vi "InitBallHandling.vi"   [LabVIEW 2023]
doc: "This VI initializes miscellaneous devices such as the compressor and any decorations."
uses:
  <vilib>/Rock Robotics/WPI/ThirdParty/Phoenix-LabVIEW/Motor Controller/Controls/CTRE_Phoenix_MotorControl_TalonFXInvertType.ctl
  <vilib>/Rock Robotics/WPI/ThirdParty/Phoenix-LabVIEW/Motor Controller/Controls/CTRE_Phoenix_MotorControl_NeutralMode.ctl
  <vilib>/Rock Robotics/WPI/ThirdParty/Phoenix-LabVIEW/Motor Controller/Controls/CTRE_Phoenix_MotorControl_FeedbackDevice_TalonFX.ctl
  <vilib>/Rock Robotics/WPI/ThirdParty/Phoenix-LabVIEW/Motor Controller/Controls/CTRE_Phoenix_MotorControl_SupplyCurrentLimitConfiguration.ctl
  <vilib>/Rock Robotics/WPI/ThirdParty/Phoenix-LabVIEW/Motor Controller/Controls/CTRE_Phoenix_MotorControl_StatusFrameEnhanced.ctl
  <vilib>/Rock Robotics/WPI/ThirdParty/Phoenix-LabVIEW/Motor Controller/Controls/CTRE_Phoenix_MotorControl_LimitSwitchSource_Local.ctl
  <vilib>/Rock Robotics/WPI/ThirdParty/Phoenix-LabVIEW/Motor Controller/Controls/CTRE_Phoenix_MotorControl_LimitSwitchNormal.ctl
  GlobalBallHandling.vi
types:
  T1 = typedef "CTRE_Phoenix_MotorControl_LimitSwitchNormal.ctl" = enum16{"Normally Open", "Normally Closed", "Disabled"}
  T2 = typedef "CTRE_Phoenix_MotorControl_LimitSwitchSource_Local.ctl" = enum16{"Feedback Connector", "Remote Talon SRX", "Remote CANifier", "Deactivated"}
  T3 = typedef "CTRE_Phoenix_MotorControl_StatusFrameEnhanced.ctl" = u16
  T4 = typedef "CTRE_Phoenix_MotorControl_SupplyCurrentLimitConfiguration.ctl" = cluster{"Enable?":bool, "Current Limit":dbl, "Threshold Current":dbl, "Threshold Time":dbl}
  T5 = typedef "CTRE_Phoenix_MotorControl_FeedbackDevice_TalonFX.ctl" = i8
  T6 = typedef "CTRE_Phoenix_MotorControl_NeutralMode.ctl" = enum8{"EEPROMSetting", "Override to Coast", "Override to Brake"}
  T7 = typedef "CTRE_Phoenix_MotorControl_TalonFXInvertType.ctl" = enum16{"Counter-Clockwise", "Clockwise"}
  T8 = typedef "WPI_MotorControlDeviceRef.ctl" = cluster{"DeviceStatus":errorcluster, "Type":T9, "PWM":cluster{"PWM Channel":T10, "DeadBand":T11}, "CAN":cluster{"Device Number":u8, "SetOutput VI Ref":variant, "GetOutput VI Ref":variant, "Enable VI Ref":variant, "Disable VI Ref":variant, "Data":variant}, "Invert":bool, "DIO PWM":cluster{"PWM \"Enable\" Channel":T10, "DIOChannel":T12, "PWM Rate":dbl}}
  T9 = typedef "WPI_MotorControlType.ctl" = enum16{"PWM", "CAN", "DIO PWM"}
  T10 = typedef "FPGA_DIOPWMChannel.ctl" = enum8{"PWM 0", "PWM 1", "PWM 2", "PWM 3", "PWM 4", "PWM 5", "PWM 6", "PWM 7", "PWM 8", "PWM 9", "PWM MXP 0", "PWM MXP 1", "PWM MXP 2", "PWM MXP 3", "PWM MXP 4", "PWM MXP 5", "PWM MXP 6", "PWM MXP 7", "PWM MXP 8", "PWM MXP 9", "Invalid"}
  T11 = typedef "WPI_PWMDeadband.ctl" = cluster{"Name":string, "maxPositivePwm":i32, "minPositivePwm":i32, "centerPwm":i32, "maxNegativePwm":i32, "minNegativePwm":i32, "angularRange":u16}
  T12 = typedef "FPGA_DIOChannel.ctl" = enum8{"DIO 0", "DIO 1", "DIO 2", "DIO 3", "DIO 4", "DIO 5", "DIO 6", "DIO 7", "DIO 8", "DIO 9", "DIO MXP 0", "DIO MXP 1", "DIO MXP 2", "DIO MXP 3", "DIO MXP 4", "DIO MXP 5", "DIO MXP 6", "DIO MXP 7", "DIO MXP 8", "DIO MXP 9", "DIO MXP 10", "DIO MXP 11", "DIO MXP 12", "DIO MXP 13", "DIO MXP 14", "DIO MXP 15", "SPI Port CS1", "SPI Port CS2", "SPI Port CS3", "SPI Port MISO", "SPI Port MOSI", "Invalid"}
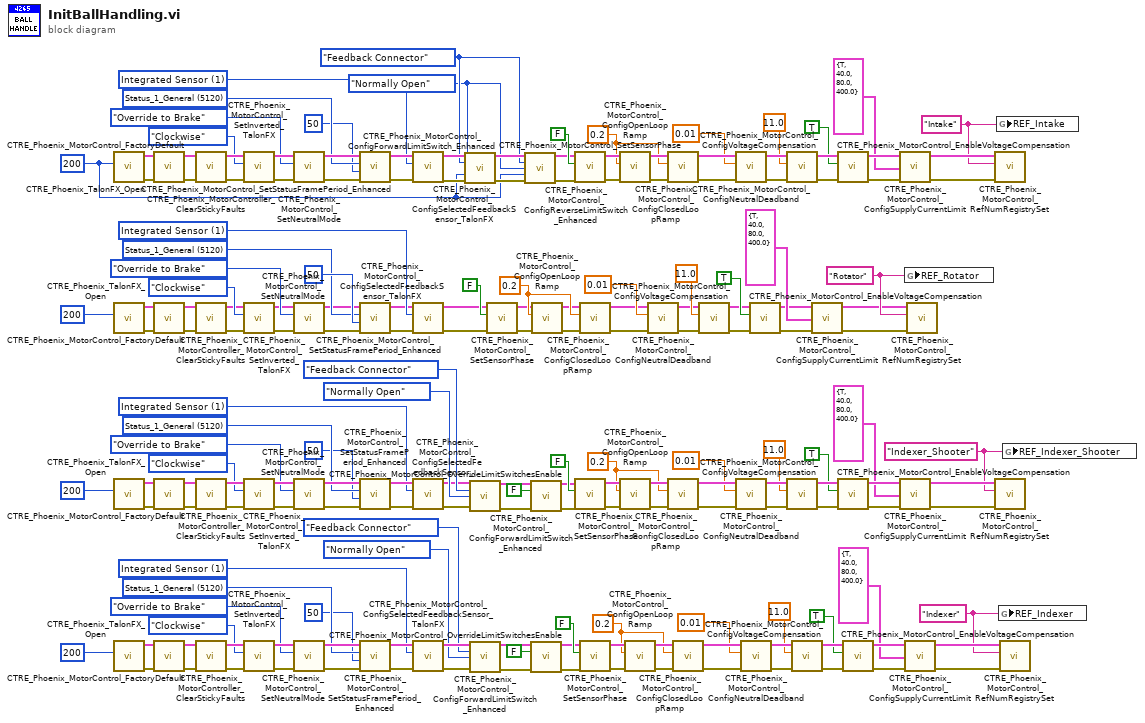
[diagram p0: block diagram]
diagram:
  w19 = T3 5120 items=["Status_1_General"=5120, "Status_2_Feedback0"=5184, "Status_3_Quadrature"=5248, "Status_4_AinTempVbat"=5312, "Status_6_Misc"=5440, "Status_7_CommStatus"=5504, "Status_8_PulseWidth"=5568, "Status_9_MotProfBuffer"=5632, "Status_10_MotionMagic"=5696, "Status_11_UartGadgeteer"=5760, "Status_12_Feedback1"=5824, "Status_13_Base_PIDF0"=5888, "Status_14_Turn_PIDF1"=5952, "Status_15_FirmwareApiStatus"=6016, "Status_Brushless_Current"=4672] ("Status Frame")
  w10 = "Indexer" ("refnum name")
  w15 = 0.2 ("secondsFromNeutralToFull")
  w17 = T5 1 items=["Integrated Sensor"=1, "Sensor Sum (S0 + S1)"=9, "Sensor Difference (D0 - D1)"=10, "Remote Source 0"=11, "Remote Source 1"=12, "None"=14, "Software Emulated"=15] ("Talon FX Feedback Device")
  w52 = CTRE_Phoenix_MotorControl_LimitSwitchNormal."Normally Open" ("NormallyOpenOrClosed")
  w53 = CTRE_Phoenix_MotorControl_LimitSwitchSource_Local."Feedback Connector" ("Limit Switch Source")
  w76 = T3 5120 items=["Status_1_General"=5120, "Status_2_Feedback0"=5184, "Status_3_Quadrature"=5248, "Status_4_AinTempVbat"=5312, "Status_6_Misc"=5440, "Status_7_CommStatus"=5504, "Status_8_PulseWidth"=5568, "Status_9_MotProfBuffer"=5632, "Status_10_MotionMagic"=5696, "Status_11_UartGadgeteer"=5760, "Status_12_Feedback1"=5824, "Status_13_Base_PIDF0"=5888, "Status_14_Turn_PIDF1"=5952, "Status_15_FirmwareApiStatus"=6016, "Status_Brushless_Current"=4672] ("Status Frame")
  w67 = "Indexer_Shooter" ("refnum name")
  w72 = 0.2 ("secondsFromNeutralToFull")
  w74 = T5 1 items=["Integrated Sensor"=1, "Sensor Sum (S0 + S1)"=9, "Sensor Difference (D0 - D1)"=10, "Remote Source 0"=11, "Remote Source 1"=12, "None"=14, "Software Emulated"=15] ("Talon FX Feedback Device")
  w137 = T3 5120 items=["Status_1_General"=5120, "Status_2_Feedback0"=5184, "Status_3_Quadrature"=5248, "Status_4_AinTempVbat"=5312, "Status_6_Misc"=5440, "Status_7_CommStatus"=5504, "Status_8_PulseWidth"=5568, "Status_9_MotProfBuffer"=5632, "Status_10_MotionMagic"=5696, "Status_11_UartGadgeteer"=5760, "Status_12_Feedback1"=5824, "Status_13_Base_PIDF0"=5888, "Status_14_Turn_PIDF1"=5952, "Status_15_FirmwareApiStatus"=6016, "Status_Brushless_Current"=4672] ("Status Frame")
  w146 = "Rotator" ("refnum name")
  w141 = 0.2 ("secondsFromNeutralToFull")
  w139 = T5 1 items=["Integrated Sensor"=1, "Sensor Sum (S0 + S1)"=9, "Sensor Difference (D0 - D1)"=10, "Remote Source 0"=11, "Remote Source 1"=12, "None"=14, "Software Emulated"=15] ("Talon FX Feedback Device")
  w156 = T3 5120 items=["Status_1_General"=5120, "Status_2_Feedback0"=5184, "Status_3_Quadrature"=5248, "Status_4_AinTempVbat"=5312, "Status_6_Misc"=5440, "Status_7_CommStatus"=5504, "Status_8_PulseWidth"=5568, "Status_9_MotProfBuffer"=5632, "Status_10_MotionMagic"=5696, "Status_11_UartGadgeteer"=5760, "Status_12_Feedback1"=5824, "Status_13_Base_PIDF0"=5888, "Status_14_Turn_PIDF1"=5952, "Status_15_FirmwareApiStatus"=6016, "Status_Brushless_Current"=4672] ("Status Frame")
  w147 = "Intake" ("refnum name")
  w152 = 0.2 ("secondsFromNeutralToFull")
  w154 = T5 1 items=["Integrated Sensor"=1, "Sensor Sum (S0 + S1)"=9, "Sensor Difference (D0 - D1)"=10, "Remote Source 0"=11, "Remote Source 1"=12, "None"=14, "Software Emulated"=15] ("Talon FX Feedback Device")
  w51 = u8 200 ("Device Number")
  n1 = call <vilib>:"CTRE_Phoenix_TalonFX_Open.vi"("Device Number"=w51) -> ("error out"=w170:errorcluster, "PhoenixMotorControlDevRef"=w177:T8)  [unwired: 9 in]
  n2 = call <vilib>:"CTRE_Phoenix_TalonFX_Open.vi"("Device Number"=u8 200) -> ("error out"=w121:errorcluster, "PhoenixMotorControlDevRef"=w113:T8)  [unwired: 9 in]
  n3 = call <vilib>:"CTRE_Phoenix_TalonFX_Open.vi"("Device Number"=u8 200) -> ("error out"=w90:errorcluster, "PhoenixMotorControlDevRef"=w98:T8)  [unwired: 9 in]
  n4 = call <vilib>:"CTRE_Phoenix_TalonFX_Open.vi"("Device Number"=u8 200) -> ("error out"=w33:errorcluster, "PhoenixMotorControlDevRef"=w41:T8)  [unwired: 9 in]
  n5 = call <vilib>:"CTRE_Phoenix_MotorControl_FactoryDefault.vi"("error in"=w170, "PhoenixMotorControlDevRef"=w177) -> ("error out"=w171:errorcluster, "PhoenixMotorControlDevRef"=w178:T8)  [unwired: 8 in]
  n6 = call <vilib>:"CTRE_Phoenix_MotorControl_FactoryDefault.vi"("error in"=w121, "PhoenixMotorControlDevRef"=w113) -> ("error out"=w120:errorcluster, "PhoenixMotorControlDevRef"=w112:T8)  [unwired: 8 in]
  n7 = call <vilib>:"CTRE_Phoenix_MotorControl_FactoryDefault.vi"("error in"=w90, "PhoenixMotorControlDevRef"=w98) -> ("error out"=w91:errorcluster, "PhoenixMotorControlDevRef"=w99:T8)  [unwired: 8 in]
  n8 = call <vilib>:"CTRE_Phoenix_MotorControl_FactoryDefault.vi"("error in"=w33, "PhoenixMotorControlDevRef"=w41) -> ("error out"=w34:errorcluster, "PhoenixMotorControlDevRef"=w42:T8)  [unwired: 8 in]
  n9 = call <vilib>:"CTRE_Phoenix_MotorController_ClearStickyFaults.vi"("error in"=w171, "PhoenixMotorControlDevRef"=w178) -> ("error out"=w172:errorcluster, "PhoenixMotorControlDevRef"=w179:T8)  [unwired: 8 in]
  n10 = call <vilib>:"CTRE_Phoenix_MotorController_ClearStickyFaults.vi"("error in"=w120, "PhoenixMotorControlDevRef"=w112) -> ("error out"=w119:errorcluster, "PhoenixMotorControlDevRef"=w111:T8)  [unwired: 8 in]
  n11 = call <vilib>:"CTRE_Phoenix_MotorController_ClearStickyFaults.vi"("error in"=w91, "PhoenixMotorControlDevRef"=w99) -> ("error out"=w92:errorcluster, "PhoenixMotorControlDevRef"=w100:T8)  [unwired: 8 in]
  n12 = call <vilib>:"CTRE_Phoenix_MotorController_ClearStickyFaults.vi"("error in"=w34, "PhoenixMotorControlDevRef"=w42) -> ("error out"=w35:errorcluster, "PhoenixMotorControlDevRef"=w43:T8)  [unwired: 8 in]
  n13 = call <vilib>:"CTRE_Phoenix_MotorControl_SetInverted_TalonFX.vi"("error in (no error)"=w172, "Invert Type"=CTRE_Phoenix_MotorControl_TalonFXInvertType."Clockwise", "PhoenixMotorControlDevRef"=w179) -> ("error out"=w173:errorcluster, "PhoenixMotorControlDevRef"=w180:T8)  [unwired: 7 in]
  n14 = call <vilib>:"CTRE_Phoenix_MotorControl_SetInverted_TalonFX.vi"("error in (no error)"=w119, "Invert Type"=CTRE_Phoenix_MotorControl_TalonFXInvertType."Clockwise", "PhoenixMotorControlDevRef"=w111) -> ("error out"=w118:errorcluster, "PhoenixMotorControlDevRef"=w110:T8)  [unwired: 7 in]
  n15 = call <vilib>:"CTRE_Phoenix_MotorControl_SetInverted_TalonFX.vi"("error in (no error)"=w92, "Invert Type"=CTRE_Phoenix_MotorControl_TalonFXInvertType."Clockwise", "PhoenixMotorControlDevRef"=w100) -> ("error out"=w93:errorcluster, "PhoenixMotorControlDevRef"=w101:T8)  [unwired: 7 in]
  n16 = call <vilib>:"CTRE_Phoenix_MotorControl_SetInverted_TalonFX.vi"("error in (no error)"=w35, "Invert Type"=CTRE_Phoenix_MotorControl_TalonFXInvertType."Clockwise", "PhoenixMotorControlDevRef"=w43) -> ("error out"=w36:errorcluster, "PhoenixMotorControlDevRef"=w44:T8)  [unwired: 7 in]
  n17 = call <vilib>:"CTRE_Phoenix_MotorControl_SetNeutralMode.vi"("error in (no error)"=w173, "Motor Control Neutral Mode"=CTRE_Phoenix_MotorControl_NeutralMode."Override to Brake", "PhoenixMotorControlDevRef"=w180) -> ("error out"=w174:errorcluster, "PhoenixMotorControlDevRef"=w184:T8)  [unwired: 7 in]
  n18 = call <vilib>:"CTRE_Phoenix_MotorControl_SetNeutralMode.vi"("error in (no error)"=w118, "Motor Control Neutral Mode"=CTRE_Phoenix_MotorControl_NeutralMode."Override to Brake", "PhoenixMotorControlDevRef"=w110) -> ("error out"=w117:errorcluster, "PhoenixMotorControlDevRef"=w106:T8)  [unwired: 7 in]
  n19 = call <vilib>:"CTRE_Phoenix_MotorControl_SetNeutralMode.vi"("error in (no error)"=w93, "Motor Control Neutral Mode"=CTRE_Phoenix_MotorControl_NeutralMode."Override to Brake", "PhoenixMotorControlDevRef"=w101) -> ("error out"=w94:errorcluster, "PhoenixMotorControlDevRef"=w105:T8)  [unwired: 7 in]
  n20 = call <vilib>:"CTRE_Phoenix_MotorControl_SetNeutralMode.vi"("error in (no error)"=w36, "Motor Control Neutral Mode"=CTRE_Phoenix_MotorControl_NeutralMode."Override to Brake", "PhoenixMotorControlDevRef"=w44) -> ("error out"=w37:errorcluster, "PhoenixMotorControlDevRef"=w48:T8)  [unwired: 7 in]
  n21 = call <vilib>:"CTRE_Phoenix_MotorControl_SetStatusFramePeriod_Enhanced.vi"("error in (no error)"=w174, "periodMs"=50, "Status Frame"=w156, "PhoenixMotorControlDevRef"=w184) -> ("error out"=w175:errorcluster, "PhoenixMotorControlDevRef"=w176:T8)  [unwired: 6 in]
  n22 = call <vilib>:"CTRE_Phoenix_MotorControl_SetStatusFramePeriod_Enhanced.vi"("error in (no error)"=w117, "periodMs"=50, "Status Frame"=w137, "PhoenixMotorControlDevRef"=w106) -> ("error out"=w116:errorcluster, "PhoenixMotorControlDevRef"=w115:T8)  [unwired: 6 in]
  n23 = call <vilib>:"CTRE_Phoenix_MotorControl_SetStatusFramePeriod_Enhanced.vi"("error in (no error)"=w94, "periodMs"=50, "Status Frame"=w76, "PhoenixMotorControlDevRef"=w105) -> ("error out"=w95:errorcluster, "PhoenixMotorControlDevRef"=w96:T8)  [unwired: 6 in]
  n24 = call <vilib>:"CTRE_Phoenix_MotorControl_SetStatusFramePeriod_Enhanced.vi"("error in (no error)"=w37, "periodMs"=50, "Status Frame"=w19, "PhoenixMotorControlDevRef"=w48) -> ("error out"=w38:errorcluster, "PhoenixMotorControlDevRef"=w39:T8)  [unwired: 6 in]
  n25 = call <vilib>:"CTRE_Phoenix_MotorControl_ConfigSelectedFeedbackSensor_TalonFX.vi"("error in (no error)"=w175, "Talon FX Feedback Device"=w154, "PhoenixMotorControlDevRef"=w176) -> ("error out"=w56:errorcluster, "PhoenixMotorControlDevRef"=w57:T8)  [unwired: 7 in]
  n26 = call <vilib>:"CTRE_Phoenix_MotorControl_ConfigSelectedFeedbackSensor_TalonFX.vi"("error in (no error)"=w116, "Talon FX Feedback Device"=w139, "PhoenixMotorControlDevRef"=w115) -> ("error out"=w127:errorcluster, "PhoenixMotorControlDevRef"=w125:T8)  [unwired: 7 in]
  n27 = call <vilib>:"CTRE_Phoenix_MotorControl_ConfigSelectedFeedbackSensor_TalonFX.vi"("error in (no error)"=w95, "Talon FX Feedback Device"=w74, "PhoenixMotorControlDevRef"=w96) -> ("error out"=w60:errorcluster, "PhoenixMotorControlDevRef"=w61:T8)  [unwired: 7 in]
  n28 = call <vilib>:"CTRE_Phoenix_MotorControl_ConfigSelectedFeedbackSensor_TalonFX.vi"("error in (no error)"=w38, "Talon FX Feedback Device"=w17, "PhoenixMotorControlDevRef"=w39) -> ("error out"=w7:errorcluster, "PhoenixMotorControlDevRef"=w8:T8)  [unwired: 7 in]
  n29 = call <vilib>:"CTRE_Phoenix_MotorControl_ConfigForwardLimitSwitch_Enhanced.vi"("PhoenixMotorControlDevRef"=w57, "Limit Switch Source"=w53, "NormallyOpenOrClosed"=w52, "deviceID"=w51, "error in (no error)"=w56) -> ("PhoenixMotorControlDevRef"=w55:T8, "error out"=w54:errorcluster)  [unwired: 9 in]
  n30 = call <vilib>:"CTRE_Phoenix_MotorControl_ConfigForwardLimitSwitch_Enhanced.vi"("PhoenixMotorControlDevRef"=w61, "Limit Switch Source"=CTRE_Phoenix_MotorControl_LimitSwitchSource_Local."Feedback Connector", "NormallyOpenOrClosed"=CTRE_Phoenix_MotorControl_LimitSwitchNormal."Normally Open", "error in (no error)"=w60) -> ("PhoenixMotorControlDevRef"=w66:T8, "error out"=w65:errorcluster)  [unwired: 10 in]
  n31 = call <vilib>:"CTRE_Phoenix_MotorControl_ConfigForwardLimitSwitch_Enhanced.vi"("PhoenixMotorControlDevRef"=w8, "Limit Switch Source"=CTRE_Phoenix_MotorControl_LimitSwitchSource_Local."Feedback Connector", "NormallyOpenOrClosed"=CTRE_Phoenix_MotorControl_LimitSwitchNormal."Normally Open", "error in (no error)"=w7) -> ("PhoenixMotorControlDevRef"=w3:T8, "error out"=w6:errorcluster)  [unwired: 10 in]
  n32 = call <vilib>:"CTRE_Phoenix_MotorControl_SetSensorPhase.vi"("error in (no error)"=w127, "PhaseSensor"=FALSE, "PhoenixMotorControlDevRef"=w125) -> ("error out"=w128:errorcluster, "PhoenixMotorControlDevRef"=w126:T8)  [unwired: 7 in]
  n33 = call <vilib>:"CTRE_Phoenix_MotorControl_ConfigReverseLimitSwitch_Enhanced.vi"("PhoenixMotorControlDevRef"=w55, "Limit Switch Source"=w53, "NormallyOpenOrClosed"=w52, "deviceID"=w51, "error in (no error)"=w54) -> ("PhoenixMotorControlDevRef"=w50:T8, "error out"=w49:errorcluster)  [unwired: 9 in]
  n34 = call <vilib>:"CTRE_Phoenix_MotorControl_OverrideLimitSwitchesEnable.vi"("PhoenixMotorControlDevRef"=w66, "Override Limit Switch Enable?"=FALSE, "error in (no error)"=w65) -> ("PhoenixMotorControlDevRef"=w58:T8, "error out"=w59:errorcluster)  [unwired: 11 in]
  n35 = call <vilib>:"CTRE_Phoenix_MotorControl_OverrideLimitSwitchesEnable.vi"("PhoenixMotorControlDevRef"=w3, "Override Limit Switch Enable?"=FALSE, "error in (no error)"=w6) -> ("PhoenixMotorControlDevRef"=w4:T8, "error out"=w5:errorcluster)  [unwired: 11 in]
  n36 = call <vilib>:"CTRE_Phoenix_MotorControl_ConfigOpenLoopRamp.vi"("error in (no error)"=w128, "secondsFromNeutralToFull"=w141, "PhoenixMotorControlDevRef"=w126) -> ("error out"=w122:errorcluster, "PhoenixMotorControlDevRef"=w109:T8)  [unwired: 7 in]
  n37 = call <vilib>:"CTRE_Phoenix_MotorControl_SetSensorPhase.vi"("error in (no error)"=w49, "PhaseSensor"=FALSE, "PhoenixMotorControlDevRef"=w50) -> ("error out"=w165:errorcluster, "PhoenixMotorControlDevRef"=w166:T8)  [unwired: 7 in]
  n38 = call <vilib>:"CTRE_Phoenix_MotorControl_SetSensorPhase.vi"("error in (no error)"=w59, "PhaseSensor"=FALSE, "PhoenixMotorControlDevRef"=w58) -> ("error out"=w85:errorcluster, "PhoenixMotorControlDevRef"=w86:T8)  [unwired: 7 in]
  n39 = call <vilib>:"CTRE_Phoenix_MotorControl_ConfigClosedLoopRamp.vi"("error in (no error)"=w122, "secondsFromNeutralToFull"=w141, "PhoenixMotorControlDevRef"=w109) -> ("error out"=w130:errorcluster, "PhoenixMotorControlDevRef"=w129:T8)  [unwired: 7 in]
  n40 = call <vilib>:"CTRE_Phoenix_MotorControl_SetSensorPhase.vi"("error in (no error)"=w5, "PhaseSensor"=FALSE, "PhoenixMotorControlDevRef"=w4) -> ("error out"=w28:errorcluster, "PhoenixMotorControlDevRef"=w29:T8)  [unwired: 7 in]
  n41 = call <vilib>:"CTRE_Phoenix_MotorControl_ConfigOpenLoopRamp.vi"("error in (no error)"=w165, "secondsFromNeutralToFull"=w152, "PhoenixMotorControlDevRef"=w166) -> ("error out"=w169:errorcluster, "PhoenixMotorControlDevRef"=w181:T8)  [unwired: 7 in]
  n42 = call <vilib>:"CTRE_Phoenix_MotorControl_ConfigOpenLoopRamp.vi"("error in (no error)"=w85, "secondsFromNeutralToFull"=w72, "PhoenixMotorControlDevRef"=w86) -> ("error out"=w89:errorcluster, "PhoenixMotorControlDevRef"=w102:T8)  [unwired: 7 in]
  n43 = call <vilib>:"CTRE_Phoenix_MotorControl_ConfigOpenLoopRamp.vi"("error in (no error)"=w28, "secondsFromNeutralToFull"=w15, "PhoenixMotorControlDevRef"=w29) -> ("error out"=w32:errorcluster, "PhoenixMotorControlDevRef"=w45:T8)  [unwired: 7 in]
  n44 = call <vilib>:"CTRE_Phoenix_MotorControl_ConfigNeutralDeadband.vi"("error in (no error)"=w130, "Percent Deadband"=0.01, "PhoenixMotorControlDevRef"=w129) -> ("error out"=w131:errorcluster, "PhoenixMotorControlDevRef"=w132:T8)  [unwired: 7 in]
  n45 = call <vilib>:"CTRE_Phoenix_MotorControl_ConfigClosedLoopRamp.vi"("error in (no error)"=w169, "secondsFromNeutralToFull"=w152, "PhoenixMotorControlDevRef"=w181) -> ("error out"=w163:errorcluster, "PhoenixMotorControlDevRef"=w164:T8)  [unwired: 7 in]
  n46 = call <vilib>:"CTRE_Phoenix_MotorControl_ConfigClosedLoopRamp.vi"("error in (no error)"=w89, "secondsFromNeutralToFull"=w72, "PhoenixMotorControlDevRef"=w102) -> ("error out"=w83:errorcluster, "PhoenixMotorControlDevRef"=w84:T8)  [unwired: 7 in]
  n47 = call <vilib>:"CTRE_Phoenix_MotorControl_ConfigClosedLoopRamp.vi"("error in (no error)"=w32, "secondsFromNeutralToFull"=w15, "PhoenixMotorControlDevRef"=w45) -> ("error out"=w26:errorcluster, "PhoenixMotorControlDevRef"=w27:T8)  [unwired: 7 in]
  n48 = call <vilib>:"CTRE_Phoenix_MotorControl_ConfigVoltageCompensation.vi"("error in (no error)"=w131, "Saturation Voltage"=11.0, "PhoenixMotorControlDevRef"=w132) -> ("error out"=w123:errorcluster, "PhoenixMotorControlDevRef"=w108:T8)  [unwired: 7 in]
  n49 = call <vilib>:"CTRE_Phoenix_MotorControl_ConfigNeutralDeadband.vi"("error in (no error)"=w163, "Percent Deadband"=0.01, "PhoenixMotorControlDevRef"=w164) -> ("error out"=w162:errorcluster, "PhoenixMotorControlDevRef"=w161:T8)  [unwired: 7 in]
  n50 = call <vilib>:"CTRE_Phoenix_MotorControl_ConfigNeutralDeadband.vi"("error in (no error)"=w83, "Percent Deadband"=0.01, "PhoenixMotorControlDevRef"=w84) -> ("error out"=w82:errorcluster, "PhoenixMotorControlDevRef"=w81:T8)  [unwired: 7 in]
  n51 = call <vilib>:"CTRE_Phoenix_MotorControl_ConfigNeutralDeadband.vi"("error in (no error)"=w26, "Percent Deadband"=0.01, "PhoenixMotorControlDevRef"=w27) -> ("error out"=w25:errorcluster, "PhoenixMotorControlDevRef"=w24:T8)  [unwired: 7 in]
  n52 = call <vilib>:"CTRE_Phoenix_MotorControl_EnableVoltageCompensation.vi"("error in (no error)"=w123, "Enable Voltage Compensation?"=TRUE, "PhoenixMotorControlDevRef"=w108) -> ("error out"=w124:errorcluster, "PhoenixMotorControlDevRef"=w107:T8)  [unwired: 7 in]
  n53 = call <vilib>:"CTRE_Phoenix_MotorControl_ConfigVoltageCompensation.vi"("error in (no error)"=w162, "Saturation Voltage"=11.0, "PhoenixMotorControlDevRef"=w161) -> ("error out"=w168:errorcluster, "PhoenixMotorControlDevRef"=w182:T8)  [unwired: 7 in]
  n54 = call <vilib>:"CTRE_Phoenix_MotorControl_ConfigVoltageCompensation.vi"("error in (no error)"=w82, "Saturation Voltage"=11.0, "PhoenixMotorControlDevRef"=w81) -> ("error out"=w88:errorcluster, "PhoenixMotorControlDevRef"=w103:T8)  [unwired: 7 in]
  n55 = call <vilib>:"CTRE_Phoenix_MotorControl_ConfigVoltageCompensation.vi"("error in (no error)"=w25, "Saturation Voltage"=11.0, "PhoenixMotorControlDevRef"=w24) -> ("error out"=w31:errorcluster, "PhoenixMotorControlDevRef"=w46:T8)  [unwired: 7 in]
  n56 = call <vilib>:"CTRE_Phoenix_MotorControl_ConfigSupplyCurrentLimit.vi"("error in (no error)"=w124, "Supply Current Limit Configuration"=T4 {"Enable?"=TRUE, "Current Limit"=40.0, "Threshold Current"=80.0, "Threshold Time"=400.0}, "PhoenixMotorControlDevRef"=w107) -> ("error out"=w134:errorcluster, "PhoenixMotorControlDevRef"=w133:T8)  [unwired: 7 in]
  n57 = call <vilib>:"CTRE_Phoenix_MotorControl_EnableVoltageCompensation.vi"("error in (no error)"=w168, "Enable Voltage Compensation?"=TRUE, "PhoenixMotorControlDevRef"=w182) -> ("error out"=w167:errorcluster, "PhoenixMotorControlDevRef"=w183:T8)  [unwired: 7 in]
  n58 = call <vilib>:"CTRE_Phoenix_MotorControl_EnableVoltageCompensation.vi"("error in (no error)"=w88, "Enable Voltage Compensation?"=TRUE, "PhoenixMotorControlDevRef"=w103) -> ("error out"=w87:errorcluster, "PhoenixMotorControlDevRef"=w104:T8)  [unwired: 7 in]
  n59 = call <vilib>:"CTRE_Phoenix_MotorControl_EnableVoltageCompensation.vi"("error in (no error)"=w31, "Enable Voltage Compensation?"=TRUE, "PhoenixMotorControlDevRef"=w46) -> ("error out"=w30:errorcluster, "PhoenixMotorControlDevRef"=w47:T8)  [unwired: 7 in]
  n60 = call <vilib>:"CTRE_Phoenix_MotorControl_ConfigSupplyCurrentLimit.vi"("error in (no error)"=w167, "Supply Current Limit Configuration"=T4 {"Enable?"=TRUE, "Current Limit"=40.0, "Threshold Current"=80.0, "Threshold Time"=400.0}, "PhoenixMotorControlDevRef"=w183) -> ("error out"=w159:errorcluster, "PhoenixMotorControlDevRef"=w160:T8)  [unwired: 7 in]
  n61 = call <vilib>:"CTRE_Phoenix_MotorControl_ConfigSupplyCurrentLimit.vi"("error in (no error)"=w87, "Supply Current Limit Configuration"=T4 {"Enable?"=TRUE, "Current Limit"=40.0, "Threshold Current"=80.0, "Threshold Time"=400.0}, "PhoenixMotorControlDevRef"=w104) -> ("error out"=w79:errorcluster, "PhoenixMotorControlDevRef"=w80:T8)  [unwired: 7 in]
  n62 = global write "GlobalBallHandling.vi" "REF_Rotator"(w146) -> ()
  n63 = call <vilib>:"CTRE_Phoenix_MotorControl_ConfigSupplyCurrentLimit.vi"("error in (no error)"=w30, "Supply Current Limit Configuration"=T4 {"Enable?"=TRUE, "Current Limit"=40.0, "Threshold Current"=80.0, "Threshold Time"=400.0}, "PhoenixMotorControlDevRef"=w47) -> ("error out"=w22:errorcluster, "PhoenixMotorControlDevRef"=w23:T8)  [unwired: 7 in]
  n64 = call <vilib>:"CTRE_Phoenix_MotorControl_RefNumRegistrySet.vi"("error in (no error)"=w134, "refnum name"=w146, "PhoenixMotorControlDevRef"=w133) -> ()  [unwired: 7 in, 2 out]
  n65 = call <vilib>:"CTRE_Phoenix_MotorControl_RefNumRegistrySet.vi"("error in (no error)"=w159, "refnum name"=w147, "PhoenixMotorControlDevRef"=w160) -> ()  [unwired: 7 in, 2 out]
  n66 = call <vilib>:"CTRE_Phoenix_MotorControl_RefNumRegistrySet.vi"("error in (no error)"=w79, "refnum name"=w67, "PhoenixMotorControlDevRef"=w80) -> ()  [unwired: 7 in, 2 out]
  n67 = global write "GlobalBallHandling.vi" "REF_Intake"(w147) -> ()
  n68 = global write "GlobalBallHandling.vi" "REF_Indexer"(w10) -> ()
  n69 = call <vilib>:"CTRE_Phoenix_MotorControl_RefNumRegistrySet.vi"("error in (no error)"=w22, "refnum name"=w10, "PhoenixMotorControlDevRef"=w23) -> ()  [unwired: 7 in, 2 out]
  n70 = global write "GlobalBallHandling.vi" "REF_Indexer_Shooter"(w67) -> ()
